vi "array_to_grayscale.vi"(4 "Y Flip":bool, 6 "max level":dbl, 8 "Y Dim":i32, 9 "X Dim":i32, 11 "Input":dbl[](array[numeric])) -> (2 "Output Array":dbl[][](array[numeric]), 3 "picture":picture)   [LabVIEW 2020]
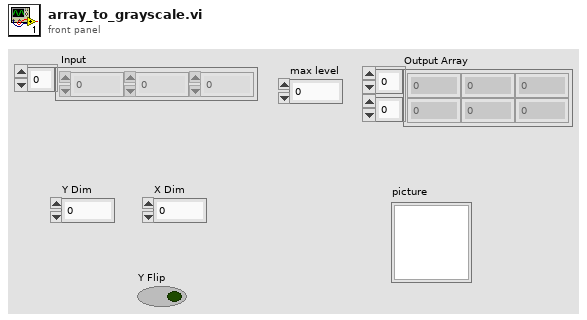
[diagram p1: front panel]
types:
  T1 = typedef "imagedata.ctl" = cluster{"image type":i32, "image depth":i32, "image":u8[], "mask":u8[], "colors":u32[], "Rectangle":cluster{"left":i16, "top":i16, "right":i16, "bottom":i16}}
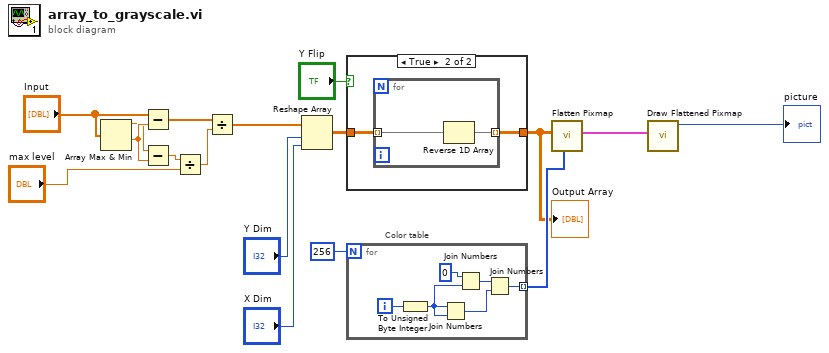
[diagram p0: block diagram]
diagram:
  # "Color table"
  n1 = Array Max & Min(array="Input") -> (max value=w1:dbl, min value=w2:dbl)  [unwired: 2 out]
  n2 = Subtract(x="Input", y=w2) -> (x-y=w3:dbl[])
  n3 = Subtract(x=w1, y=w2) -> (x-y=w4:dbl)
  n4 = Divide(x=w4, y="max level") -> (x/y=w5:dbl)
  n5 = Divide(x=w3, y=w5) -> (x/y=w15:dbl[])
  n6 = Reshape Array(w15, "Y Dim", "X Dim") -> (w7:dbl[][])
  n7 = case shown="True" "Y Flip" {
    tunnel: w7 -> [w18 w20]
    tunnel: [w18 w19] -> w6
    frame False {
    }
    frame True {
      n8 = for {
        tunnel: w20 -> [w22] mode=indexing
        tunnel: [w21] -> w19 mode=indexing
        n9 = Reverse 1D Array(array=w22) -> (reversed array=w21:dbl[])
      }
    }
  }
  "Output Array" <- w6
  n10 = for {
    N: 256 -> [_]
    tunnel: [w23] -> w11 mode=indexing
    i -> [w28]
    n11 = To Unsigned Byte Integer(number=w28) -> (unsigned 8bit integer=w27:u8)
    n12 = Join Numbers(hi=w27, lo=w27) -> ((hi.lo)=w24:u16)
    n13 = Join Numbers(hi=u8 0, lo=w27) -> ((hi.lo)=w25:u16)
    n14 = Join Numbers(hi=w25, lo=w24) -> ((hi.lo)=w23:u32)
  }
  n15 = call <vilib>:"Flatten Pixmap.vi"("colors"=w11, "8-bit pixmap"=w6) -> ("image data"=w10:T1)  [unwired: 9 in]
  n16 = call <vilib>:"Draw Flattened Pixmap.vi"("image data"=w10) -> ("new picture"=→"picture":picture)  [unwired: 8 in]
